vi "extract initial parameters.vi"(8 "error in (no error)":errorcluster, 10 "data in":dbl[](array[numeric]), 11 "LineCCD in":refnum<class "LineCCD.lvclass">) -> (0 "error out":errorcluster, 2 "data out (copy)":dbl[](array[numeric]), 3 "LineCCD out":refnum<class "LineCCD.lvclass">)   [LabVIEW 2012, in "LineCCD.lvclass"]
uses:
  LineCCD.lvclass
  LineCCD.lvclass/LineCCD.ctl
  <vilib>/Analysis/baseanly.llb/Mean (DBL).vi
  <vilib>/Analysis/NI_AALBase.lvlib
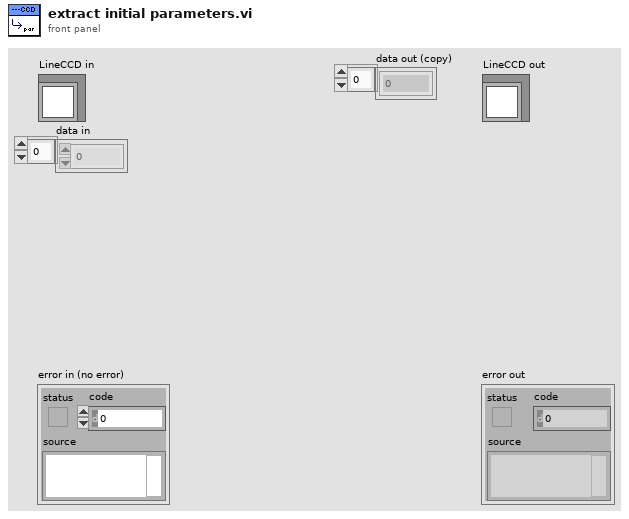
[diagram p1: front panel]
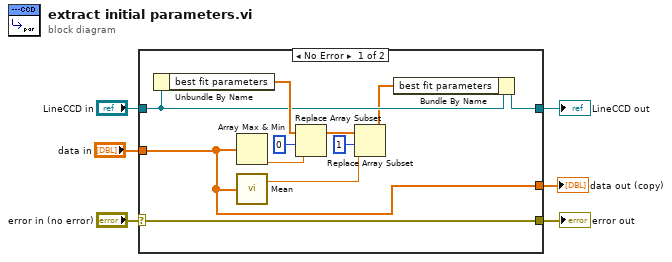
[diagram p0: block diagram]
diagram:
  n1 = case shown="No Error" "error in (no error)" {
    selector: "error in (no error)" -> [w17 w19]
    tunnel: [w17 w19] -> w5
    tunnel: [w9 w18] -> w3
    tunnel: "LineCCD in" -> [w10 w18]
    tunnel: "data in" -> [w7 _]
    tunnel: [w7 _] -> w1
    frame No Error {
      n2 = Unbundle By Name(w10) -> ("best fit parameters"=w12:dbl[])
      n3 = Array Max & Min(array=w7) -> (min value=w15:dbl)  [unwired: 3 out]
      n4 = call-poly <vilib>:"Mean.vi"("X"=w7) -> ("mean"=w16:dbl)  [unwired: 1 out]
      n5 = Replace Array Subset(array=w12, new element=w15, index=0) -> (w11:dbl[])
      n6 = Replace Array Subset(array=w11, new element=w16, index=1) -> (w8:dbl[])
      n7 = Bundle By Name(cluster=w10, "best fit parameters"=w8) -> (w9:refnum<class "LineCCD.lvclass">)
    }
    frame Error {
    }
  }
  "error out" <- w5
  "LineCCD out" <- w3
  "data out (copy)" <- w1
